vi "Create Task.vi"(8 "error in":errorcluster, 10 "Task Name":string="DigitalOutputTask", 11 "NI Digital Output in":refnum<class "NI Digital Output.lvclass">) -> (0 "error out":errorcluster, 3 "NI Digital Output out":refnum<class "NI Digital Output.lvclass">)   [LabVIEW 2023, in "HardwareAbstractionLayer_LVOOP.lvlib" / "NI Digital Output.lvclass"]
doc: "This VI DAQmx Create Auto Task"
uses:
  NI Digital Output.lvclass
  NI Digital Output.lvclass/NI Digital Output.ctl
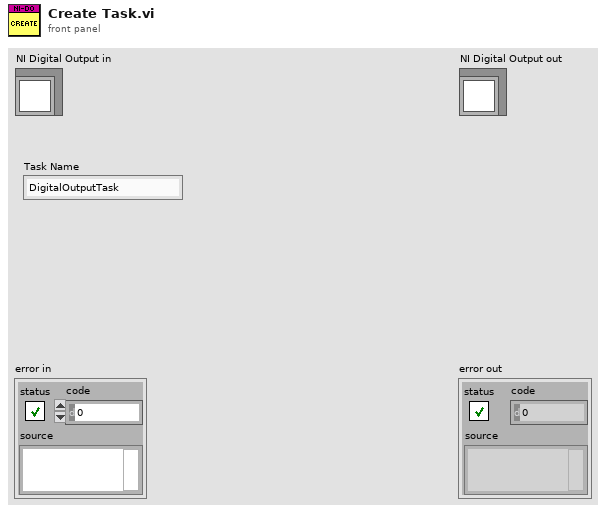
[diagram p1: front panel]
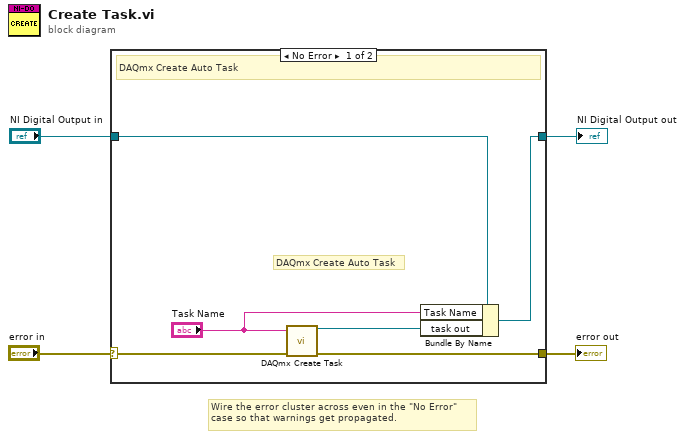
[diagram p0: block diagram]
diagram:
  # "Wire the error cluster across even in the \"No Error\"\ncase so that warnings get propagated."
  n1 = case shown="No Error" "error in" {
    selector: "error in" -> [w10 w12]
    tunnel: [w9 w12] -> w3
    tunnel: [w7 w11] -> w1
    tunnel: "NI Digital Output in" -> [w8 w11]
    frame No Error {
      # "DAQmx Create Auto Task"
      # "DAQmx Create Auto Task"
      n2 = call <vilib>:"DAQmx Create Task.vi"("new task name"="Task Name", "error in"=w10) -> ("task out"=w6:refnum<k21>, "error out"=w9:errorcluster)  [unwired: 12 in]
      n3 = Bundle By Name(cluster=w8, "Task Name"="Task Name", "task out"=w6) -> (w7:refnum<class "NI Digital Output.lvclass">)
    }
    frame Error {
    }
  }
  "error out" <- w3
  "NI Digital Output out" <- w1
